vi "servo_return_block_sequence.vi"(0 "servo 3":u8) -> ()   [LabVIEW 2017]
uses:
  GlobalVar.vi
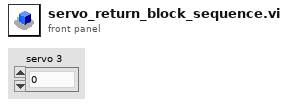
[diagram p1: front panel]
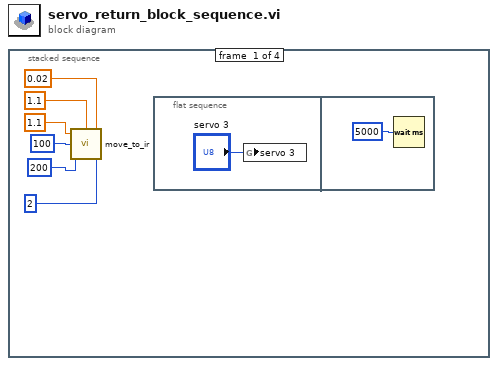
[diagram p0: block diagram]
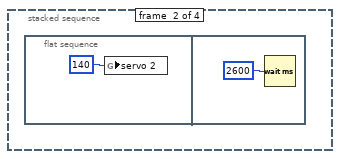
[diagram p2: hidden frame]
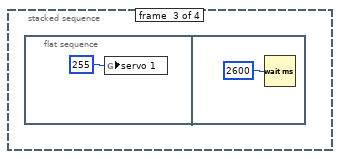
[diagram p3: hidden frame]
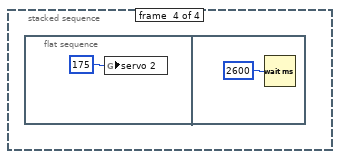
[diagram p4: hidden frame]
diagram:
  n1 = stacked-sequence {
    frame #0 {
      n2 = call "move_to_ir.vi"("step"=2, "precision"=0.02, "target_ir_r"=1.1 ("target_ir_l"), "samples"=200, "delay_after"=u32 100, "target_ir_l"=1.1) -> ()
      n3 = flat-sequence {
        frame #0 {
          n4 = global write "GlobalVar.vi" "servo 3"("servo 3") -> ()
        }
        frame #1 {
          n5 = Wait (ms)(milliseconds to wait=u32 5000) -> ()  [unwired: 1 out]
        }
      }
    }
    frame #1 {
      n6 = flat-sequence {
        frame #0 {
          n7 = global write "GlobalVar.vi" "servo 2"(u8 140 ("servo 1")) -> ()
        }
        frame #1 {
          n8 = Wait (ms)(milliseconds to wait=u32 2600) -> ()  [unwired: 1 out]
        }
      }
    }
    frame #2 {
      n9 = flat-sequence {
        frame #0 {
          n10 = global write "GlobalVar.vi" "servo 1"(u8 255 ("servo 1")) -> ()
        }
        frame #1 {
          n11 = Wait (ms)(milliseconds to wait=u32 2600) -> ()  [unwired: 1 out]
        }
      }
    }
    frame #3 {
      n12 = flat-sequence {
        frame #0 {
          n13 = global write "GlobalVar.vi" "servo 2"(u8 175 ("servo 1")) -> ()
        }
        frame #1 {
          n14 = Wait (ms)(milliseconds to wait=u32 2600) -> ()  [unwired: 1 out]
        }
      }
    }
  }
